vi "Initialize.vi"(7 "Serial Configuration":T1={"Baud Rate"=9600, "Parity"=0, "Stop Bits"=10, "Flow Control"=0} {"Flow Control" items=["None", "XON/XOFF", "RTS/CTS", "XON/XOFF & RTS/CTS", "DTR/DSR", "XON/XOFF & DTR/DSR"]; "Stop Bits" items=["1.0"=10, "1.5"=15, "2.0"=20]; "Parity" items=["None", "Odd", "Even", "Mark", "Space"]; "Baud Rate" items=["300"=300, "600"=600, "1200"=1200, "2400"=2400, "4800"=4800, "9600"=9600, "19200"=19200]}, 8 "error in (no error)":errorcluster, 9 "Reset? (T: Yes)":bool, 10 "ID Query? (T: Yes)":bool, 11 "VISA resource name":refnum<visa-resource-name>) -> (0 "error out":errorcluster, 3 "VISA resource name out":refnum<visa-resource-name>)   [LabVIEW 2018, in "Tektronix TDS 200 1000 2000 Series.lvlib"]
doc: "Establishes communication with the instrument and optionally performs an instrument identification query and/or an instrument reset. It also places the instrument in a default state needed for other instrument driver operations. Therefore, call this VI before calling other instrument driver VIs for this instrument. Generally, you need to call the <B>Initialize VI</B> only once at the beginning of an application."
uses:
  Tektronix TDS 200 1000 2000 Series.lvlib
panel:
  # "(C) 2009-2015 National Instruments.  ALL RIGHTS RESERVED."
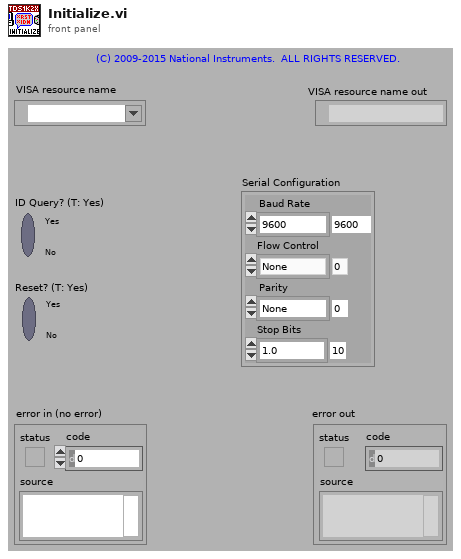
[diagram p1: front panel]
types:
  T1 = cluster{"Baud Rate":u32, "Parity":u16, "Stop Bits":u16, "Flow Control":u16}
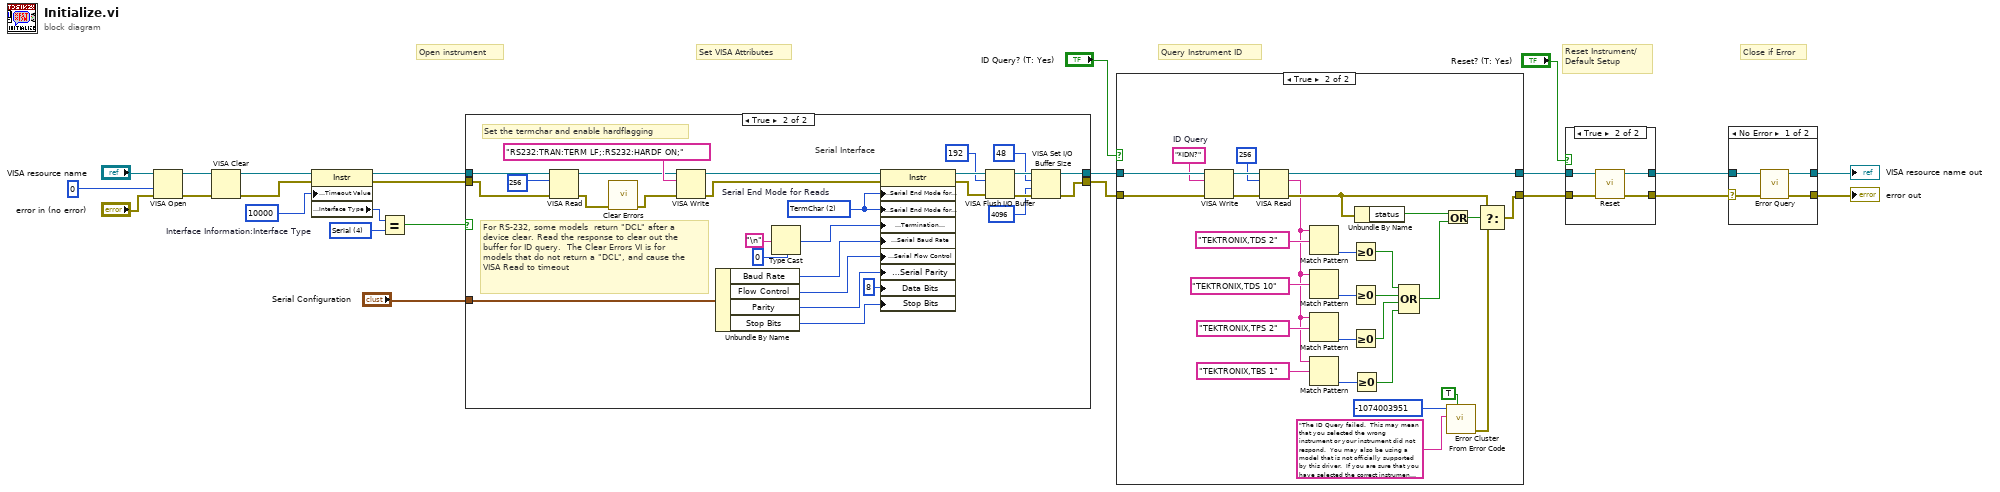
[diagram p0: block diagram]
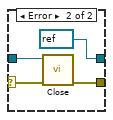
[diagram p3: hidden frame]
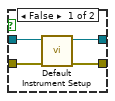
[diagram p4: hidden frame]
diagram:
  w11 = u16 4 items=["GPIB"=1, "VXI"=2, "GPIB-VXI"=3, "Serial"=4, "PXI"=5, "TCPIP"=6, "USB"=7]  # Interface Information:Interface Type
  # "Set VISA Attributes"
  # "Close if Error"
  # "Query Instrument ID"
  # "Reset Instrument/\nDefault Setup"
  # "Open instrument"
  n1 = VISA Open(access mode=u32 0, error in (no error)="error in (no error)", VISA resource name="VISA resource name") -> (VISA resource name=w9:refnum<visa-resource-name>, error out=w8:errorcluster)  [unwired: 2 out]
  n2 = VISA Clear(VISA resource name=w9, error in (no error)=w8) -> (VISA resource name out=w3:refnum<visa-resource-name>, error out=w2:errorcluster)
  n3 = property class="Instr"(reference=w3, error in=w2, "General Settings:Timeout Value"=u32 10000) -> (reference out=w14:refnum<visa-resource-name>, error out=w13:errorcluster, "Interface Information:Interface Type"=w18:u16)
  n4 = Equal?(x=w18, y=w11) -> (x = y?=w12:bool)
  n5 = case shown="True" w12 {
    tunnel: [w25 w53] -> w16
    tunnel: [w26 w50] -> w15
    tunnel: w14 -> [w25 w32]
    tunnel: w13 -> [w26 w31]
    tunnel: "Serial Configuration" -> [_ w27]
    frame False {
      # "GPIB Interface"
    }
    frame True {
      w43 = u16 2 items=["None", "LastBit", "TermChar"]  # Serial End Mode for Reads
      # "For RS-232, some models  return \"DCL\" after a device clear. Read the response to clear out the buffer for ID query.  The Clear Errors VI is for models that do not return a \"DCL\", and cause the VISA Read to timeout"
      # "Set the termchar and enable hardflagging"
      # "Serial Interface"
      n6 = VISA Read(VISA resource name=w32, byte count=u32 256, error in (no error)=w31) -> (VISA resource name out=w30:refnum<visa-resource-name>, error out=w29:errorcluster)  [unwired: 2 out]
      n7 = call "Clear Errors.vi"("error in (no error)"=w29) -> ("error out"=w28:errorcluster)  [unwired: 1 in, 5 out]
      n8 = VISA Write(VISA resource name=w30, write buffer="RS232:TRAN:TERM LF;:RS232:HARDF ON;", error in (no error)=w28) -> (VISA resource name out=w38:refnum<visa-resource-name>, error out=w37:errorcluster)  [unwired: 1 out]
      n9 = Unbundle By Name(w27) -> ("Baud Rate"=w41:u32, "Flow Control"=w39:u16, "Parity"=w40:u16, "Stop Bits"=w35:u16)
      n10 = Type Cast(type=u8 0, x="\n" ("Line Feed Constant")) -> (*(type *) &x=w42:u8)
      n11 = property class="Instr"(reference=w38, error in=w37, "Serial Settings:Serial End Mode for Reads"=w43, "Serial Settings:Serial End Mode for Writes"=w43, "Message Based Settings:Termination Character"=w42, "Serial Settings:Serial Baud Rate"=w41, "Serial Settings:Serial Flow Control"=w39, "Serial Settings:Serial Parity"=w40, "Data Bits"=u16 8 ("Serial Settings:Serial Data Bits"), "Stop Bits"=w35) -> (reference out=w49:refnum<visa-resource-name>, error out=w52:errorcluster)
      n12 = VISA Flush I/O Buffer(VISA resource name=w49, mask (16)=u16 192, error in (no error)=w52) -> (VISA resource name out=w54:refnum<visa-resource-name>, error out=w51:errorcluster)
      n13 = VISA Set I/O Buffer Size(VISA resource name=w54, mask (16)=u16 48, size (4096)=u32 4096 ("size (0)"), error in (no error)=w51) -> (VISA resource name out=w53:refnum<visa-resource-name>, error out=w50:errorcluster)
    }
  }
  n14 = case shown="True" "ID Query? (T: Yes)" {
    tunnel: [w55 w85] -> w23
    tunnel: [w56 w82] -> w24
    tunnel: w16 -> [w56 w83]
    tunnel: w15 -> [w55 w84]
    frame False {
    }
    frame True {
      w77 = "*IDN?"  # ID Query
      n15 = VISA Write(VISA resource name=w83, write buffer=w77, error in (no error)=w84) -> (VISA resource name out=w81:refnum<visa-resource-name>, error out=w80:errorcluster)  [unwired: 1 out]
      n16 = VISA Read(VISA resource name=w81, byte count=u32 256, error in (no error)=w80) -> (VISA resource name out=w82:refnum<visa-resource-name>, read buffer=w60:string, error out=w71:errorcluster)  [unwired: 1 out]
      n17 = Match Pattern(string=w60, regular expression="TEKTRONIX,TDS 2") -> (offset past match=w70:i32)  [unwired: 4 out]
      n18 = Match Pattern(string=w60, regular expression="TEKTRONIX,TDS 10") -> (offset past match=w69:i32)  [unwired: 4 out]
      n19 = Match Pattern(string=w60, regular expression="TEKTRONIX,TPS 2") -> (offset past match=w63:i32)  [unwired: 4 out]
      n20 = Match Pattern(string=w60, regular expression="TEKTRONIX,TBS 1") -> (offset past match=w58:i32)  [unwired: 4 out]
      n21 = Greater Or Equal To 0?(x=w70) -> (x >= 0?=w68:bool)
      n22 = Greater Or Equal To 0?(x=w69) -> (x >= 0?=w67:bool)
      n23 = Greater Or Equal To 0?(x=w63) -> (x >= 0?=w62:bool)
      n24 = Greater Or Equal To 0?(x=w58) -> (x >= 0?=w57:bool)
      n25 = Unbundle By Name(w71) -> ("status"=w61:bool)
      n26 = Compound Arithmetic op=OR(w68, w67, w62, w57) -> (w65:bool)
      n27 = Or(x=w61, y=w65) -> (x .or. y?=w66:bool)
      n28 = call "Error Cluster From Error Code.vi"("show call chain? (False)"=TRUE, "error message (\"\")"="The ID Query failed.  This may mean that you selected the wrong instrument or your instrument did not respond.  You may also be using a model that is not officially supported by this driver.  If you are sure that you have selected the correct instrument and it is responding, try disabling the ID Query." ("Source (VI Name)"), "error code (0)"=-1074003951 ("Code")) -> ("error out"=w76:errorcluster)  [unwired: 1 in, 5 out]
      n29 = Select(t=w71, s=w66, f=w76) -> (s? t:f=w85:errorcluster)
    }
  }
  n30 = case shown="True" "Reset? (T: Yes)" {
    tunnel: w23 -> [w88 w90]
    tunnel: [w87 w93] -> w4
    tunnel: w24 -> [w89 w91]
    tunnel: [w86 w92] -> w5
    frame False {
      n31 = call "Default Instrument Setup.vi"("error in (no error)"=w88, "VISA resource name"=w89) -> ("error out"=w87:errorcluster, "VISA resource name out"=w86:refnum<visa-resource-name>)  [unwired: 8 out]
    }
    frame True {
      n32 = call "Reset.vi"("error in (no error)"=w90, "VISA resource name"=w91) -> ("error out"=w93:errorcluster, "VISA resource name out"=w92:refnum<visa-resource-name>)  [unwired: 8 out]
    }
  }
  n33 = case shown="No Error" w4 {
    selector: w4 -> [w95 w99]
    tunnel: w5 -> [w94 w100]
    tunnel: [w97 refnum<visa-resource-name> refnum ("VISA resource name out")] -> w7
    tunnel: [w96 w101] -> w6
    frame No Error {
      n34 = call "Error Query.vi"("error in (no error)"=w95, "VISA resource name"=w94) -> ("error out"=w96:errorcluster, "VISA resource name out"=w97:refnum<visa-resource-name>)  [unwired: 8 out]
    }
    frame Error {
      n35 = call "Close.vi"("error in (no error)"=w99, "VISA resource name"=w100) -> ("error out"=w101:errorcluster)  [unwired: 9 out]
    }
  }
  "VISA resource name out" <- w7
  "error out" <- w6
